vi "Encoder.vi"(8 "Phase B":bool, 9 "Phase A":bool, 11 "CNTL":u8 format="%08b") -> (0 "STAT":u8 format="%08b", 3 "CNTR":u32)   [LabVIEW 2013]
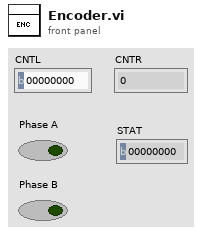
[diagram p1: front panel]
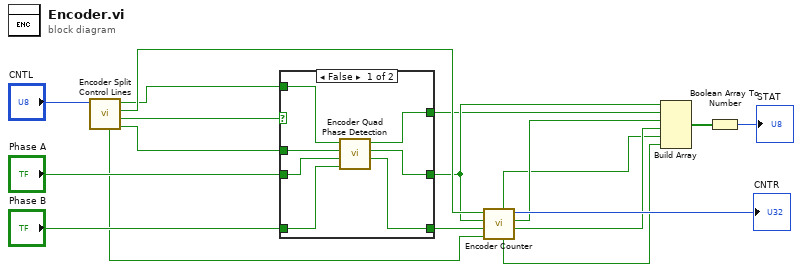
[diagram p0: block diagram]
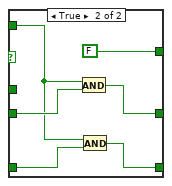
[diagram p2: hidden frame]
diagram:
  n1 = call "Encoder Split Control Lines.vi"("Control"="CNTL") -> ("Clear Error?"=w8:bool, "Dir/Clock Mode?"=w16:bool, "Reset?"=w14:bool, "Enable?"=w9:bool, "Clear Overflow?"=w4:bool)  [unwired: 6 in]
  n2 = case shown="False" w16 {
    tunnel: "Phase A" -> [w24 w31]
    tunnel: "Phase B" -> [w23 w30]
    tunnel: w9 -> [w25 w29]
    tunnel: [w20 FALSE ("Error")] -> w12
    tunnel: [w21 w27] -> w13
    tunnel: [w22 w26] -> w15
    tunnel: w8 -> [w19 _]
    frame False {
      n3 = call "Encoder Quad Phase Detection.vi"("Phase B"=w23, "Phase A"=w24, "Clear Error?"=w19, "Enable?"=w25) -> ("Signal"=w22:bool, "Backward?"=w21:bool, "Error"=w20:bool)  [unwired: 5 in]
    }
    frame True {
      n4 = And(x=w29, y=w31) -> (x .and. y?=w27:bool)
      n5 = And(x=w29, y=w30) -> (x .and. y?=w26:bool)
    }
  }
  n6 = call "Encoder Counter.vi"("Clear Overflow?"=w4, "Signal"=w15, "Backward?"=w13, "Reset?"=w14) -> ("Crossed Halfway?"=w3:bool, "Wrapped around?"=w5:bool, "Count Value"=→"CNTR":u32, "Crossed Halfway twice?"=w1:bool, "Wrapped around twice?"=w2:bool)  [unwired: 3 in]
  n7 = Build Array(w13, w12, w5, w3, w2, w1) -> (w11:bool[])
  n8 = Boolean Array To Number(Boolean array=w11) -> (number=→"STAT":u8)
